vi "Get Tab Control Refs.vi"(10 "Page Index":i32=-1, 11 "TabControl in":refnum<vi>) -> (3 "ControlsOnPage":refnum<vi>[](array[refnum]))   [LabVIEW 2017]
doc: "Return an array of the references to all control and indicators within the top level of the specified page. If index is -1, return reference to controls on all pages."
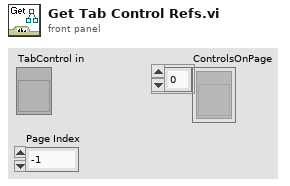
[diagram p1: front panel]
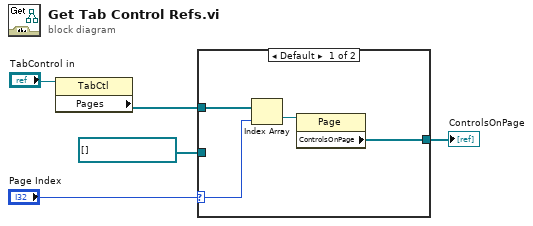
[diagram p0: block diagram]
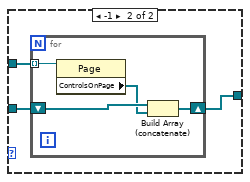
[diagram p2: hidden frame]
diagram:
  n1 = property class="TabCtl"(reference="TabControl in") -> ("Pages"=w3:refnum<vi>[])  [unwired: 1 in, 2 out]
  n2 = case shown="Default" "Page Index" {
    selector: "Page Index" -> [w6 _]
    tunnel: [w9 w10] -> w5
    tunnel: w3 -> [w7 w12]
    tunnel: refnum<vi>[] [] -> [_ w11]
    frame Default {
      n3 = Index Array(array=w7, index=w6) -> (element=w8:refnum<vi>)
      n4 = property class="Page"(reference=w8) -> ("ControlsOnPage"=w9:refnum<vi>[])  [unwired: 1 in, 2 out]
    }
    frame -1 {
      n5 = for {
        tunnel: w12 -> [w16] mode=indexing
        shift-right: [w15] -> w10
        shift-left: w11 -> [w14]
        n6 = property class="Page"(reference=w16) -> ("ControlsOnPage"=w13:refnum<vi>[])  [unwired: 1 in, 2 out]
        n7 = Build Array (concatenate)(w14, w13) -> (w15:refnum<vi>[])
      }
    }
  }
  "ControlsOnPage" <- w5
